vi "Test Executive - 副本.vi"() -> ()   [LabVIEW 2020]
uses:
  Library - Test Executive.llb/Test Executive - Globals.vi
  Library - Test Executive.llb/Test Executive.lvlib
panel:
  in  "Tab Control":T1(tab)
  in  "Serial Number":string
  out "Sequence":string
  out "Report Text":string
  in  "Operator":string
  in  "Save Report":bool
  in  "Clear Report Text":bool
  out "Sequence Name":string="None"
  in  "Abort Button":bool
  in  "Sequence Run":bool
  in  "Sequence Load":bool
  in  "Results Analyser":bool
  in  "Power Down":bool
  in  "Power Up":bool
  in  "Test":u16(ring) items=["1 Current Consumption", "2 Firmware Revision", "3 Indicators", "4 Gain", "5 Sensitivity"]
  in  "Check Test Equipment":bool
  out "errors":errorcluster
  in  "Power Down":bool
  in  "Power Up":bool
  in  "Reset All":bool
  in  "Run Single Test":bool
  out "Help Text":string="This is some help text\n"
  out "Abort":bool
  out "Error":bool
  out "Running":bool
  in  "Quit":bool
  # "Sequence"
  # "Progress"
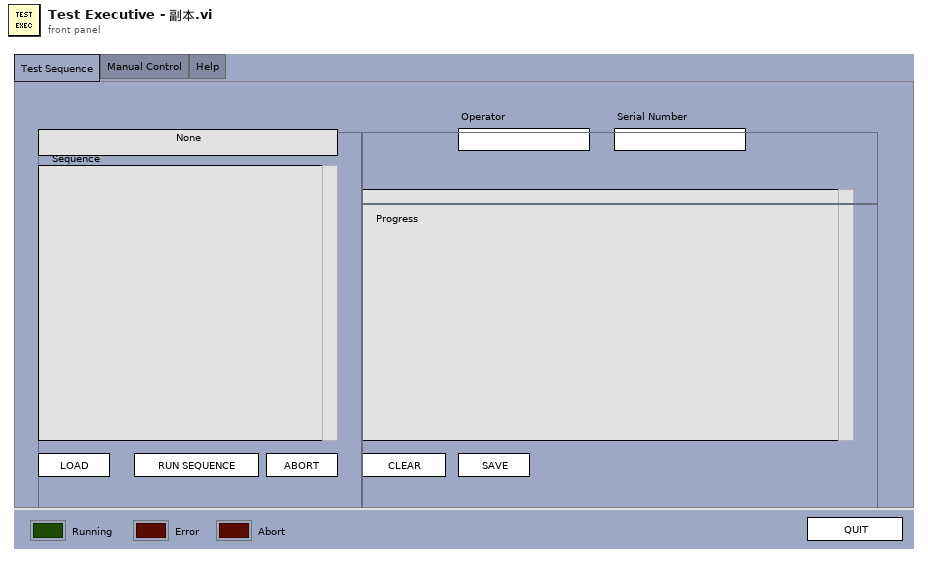
[diagram p1: front panel]
types:
  T1 = enum32{"Test Sequence", "Manual Control", "Help"}
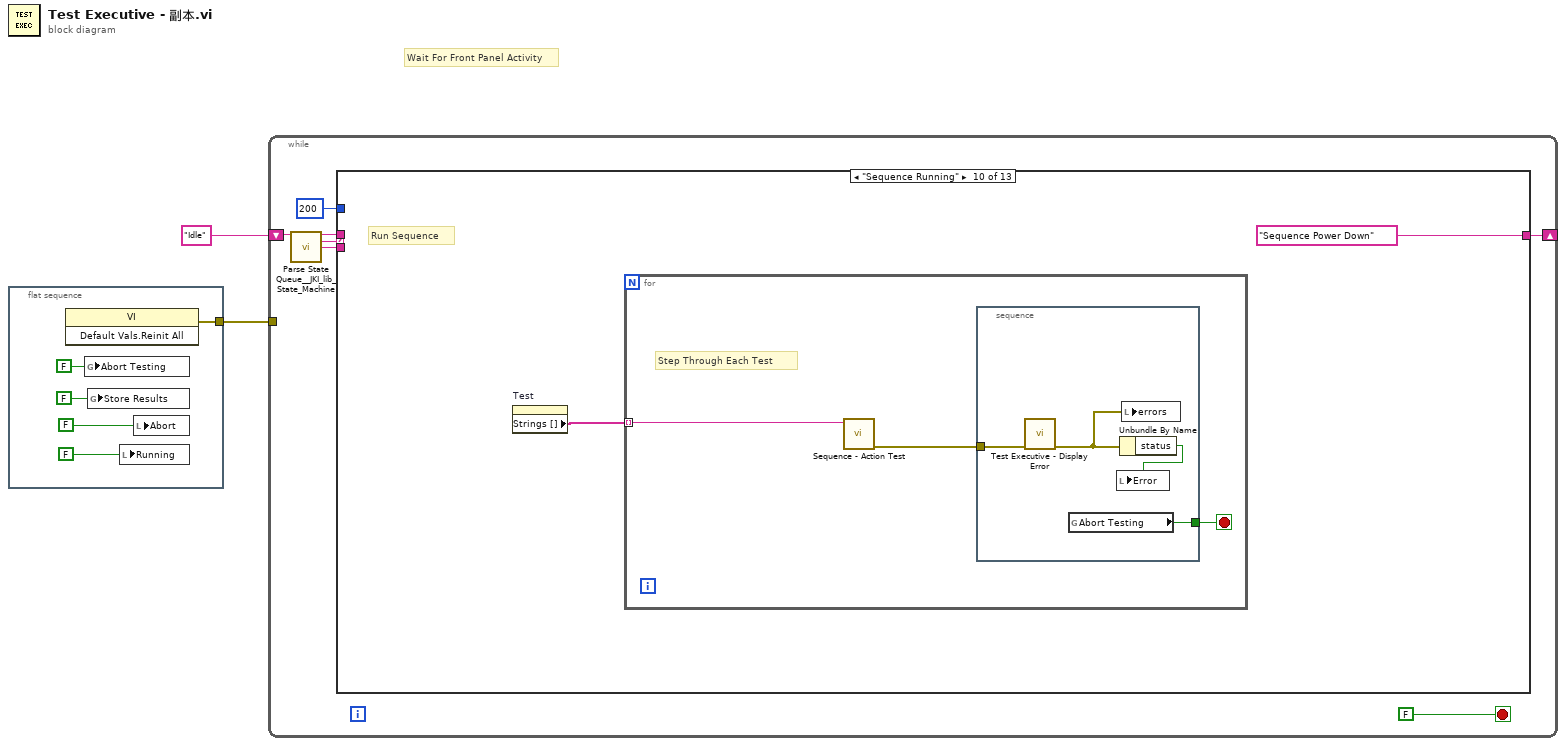
[diagram p0: block diagram]
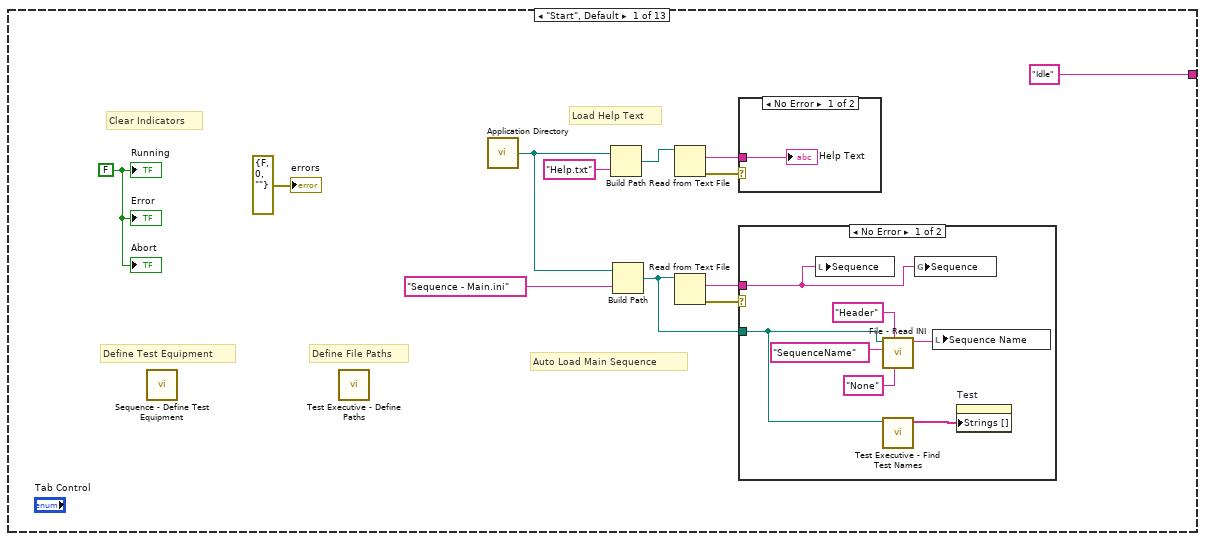
[diagram p2: hidden frame]
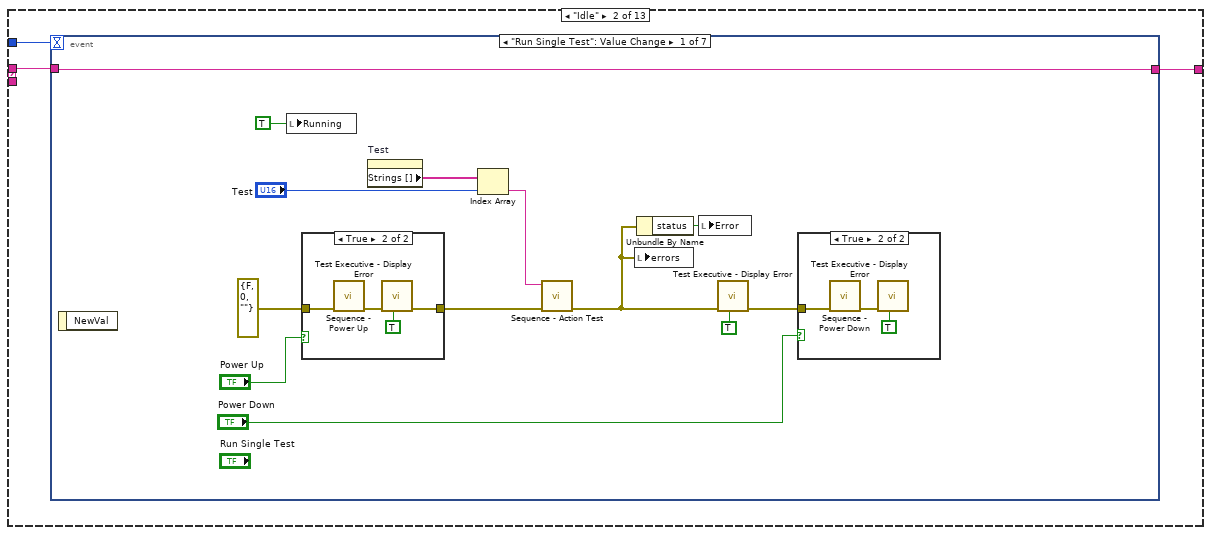
[diagram p5: hidden frame]
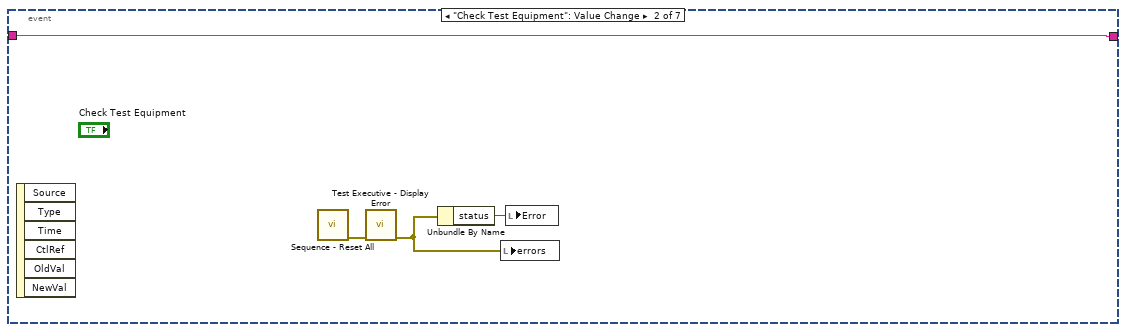
[diagram p8: hidden frame]
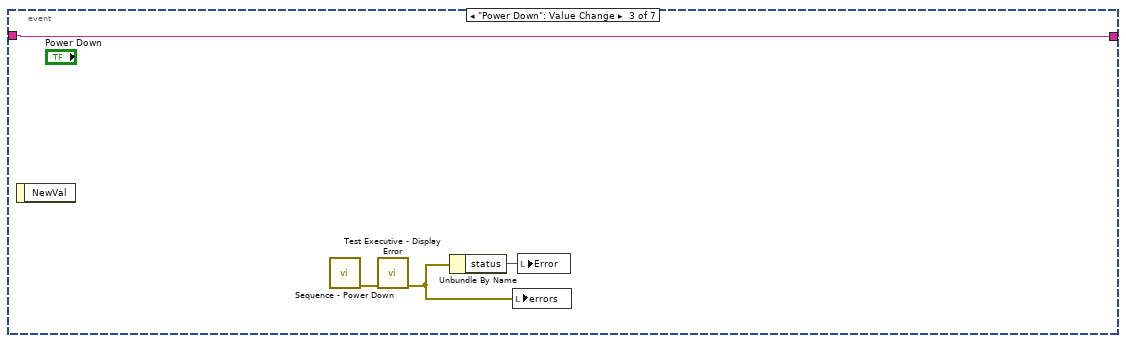
[diagram p9: hidden frame]
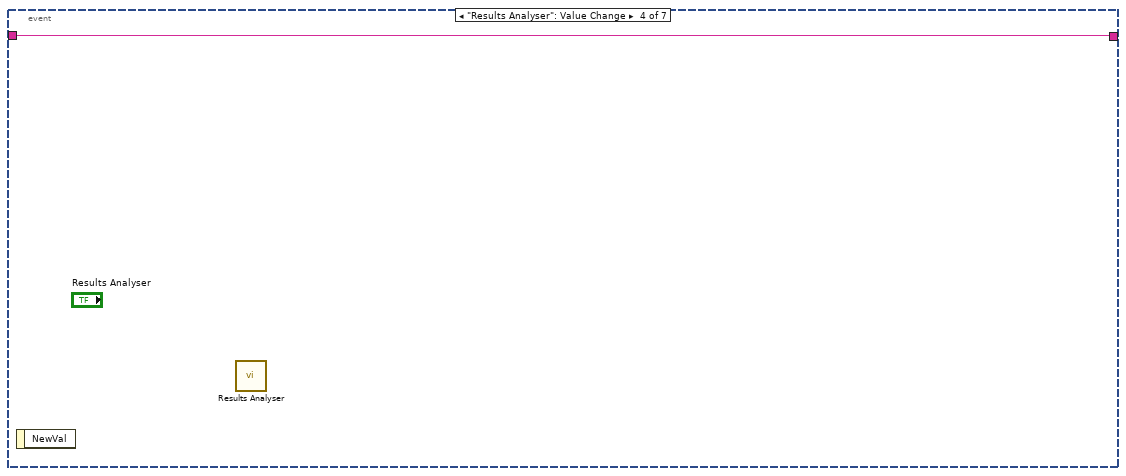
[diagram p10: hidden frame]
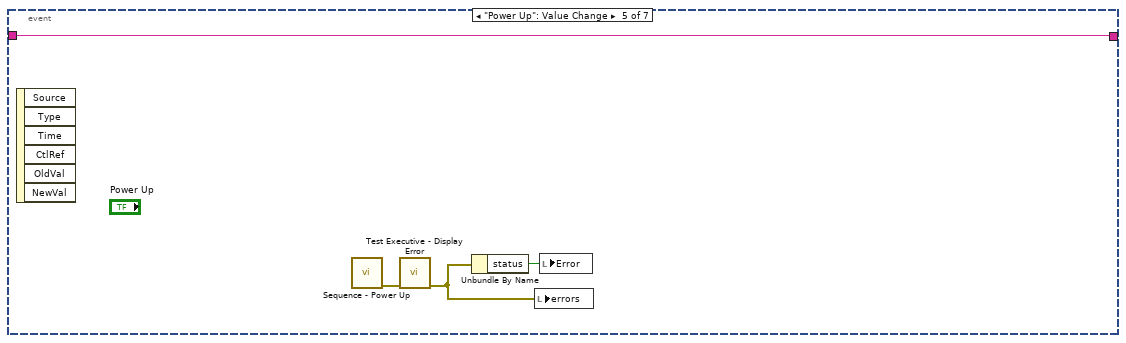
[diagram p11: hidden frame]
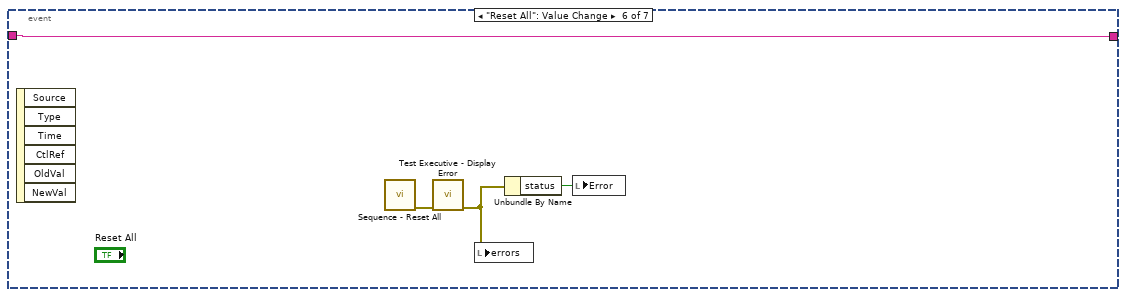
[diagram p12: hidden frame]
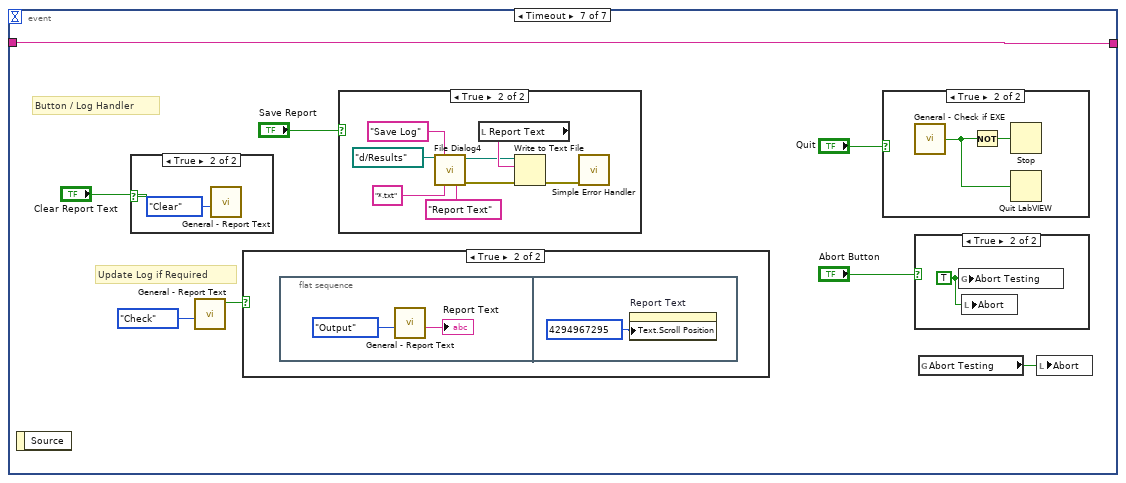
[diagram p13: hidden frame]
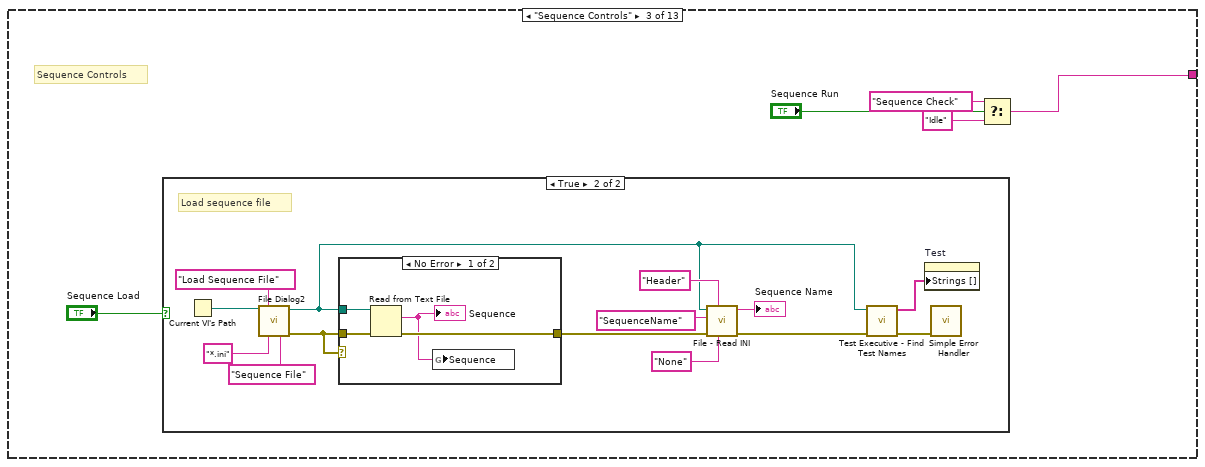
[diagram p19: hidden frame]
diagram:
  # "Wait For Front Panel Activity"
  n1 = flat-sequence {
    tunnel: [w7] -> w2
    frame #0 {
      n2 = invoke class="VI" method="Default Vals.Reinit All"() -> (error out=w7:errorcluster)  [unwired: 3 in, 2 out]
      n3 = global write "Test Executive - Globals.vi" "Abort Testing"(FALSE ("Abort Testing")) -> ()
      n4 = global write "Test Executive - Globals.vi" "Store Results"(FALSE ("Abort Testing")) -> ()
      n5 = local write "Running"(FALSE ("Abort")) -> ()
      n6 = local write "Abort"(FALSE ("Abort")) -> ()
    }
  }
  n7 = while {
    shift-right: [w13] -> _
    shift-left: "Idle" -> [w12]
    tunnel: w2 -> [_]
    stop <- FALSE stop-if-true
    n8 = call <vilib>:"Parse State Queue__JKI_lib_State_Machine.vi"("State Queue"=w12) -> ("Remaining States"=w9:string, "Current State"=w11:string, "Arguments"=w10:string)  [unwired: 12 in]
    n9 = case shown="\"Sequence Running\"" w11 {
      tunnel: ["Idle" w37 w101 w123 w131 w162 "Sequence Pre-Run" ("f") "Sequence Power Up" ("f") "Sequence Running" ("f") "Sequence Power Down" ("f") "Sequence Pass Fail" ("f") "Sequence Store Results" ("f") "Idle" ("f")] -> w13
      tunnel: w10 -> [_ _ _ _ _ _ _ _ _ _ _ _ _]
      tunnel: w9 -> [_ w36 _ _ _ _ _ _ _ _ _ _ _]
      tunnel: 200 -> [_ w35 _ _ _ _ _ _ _ _ _ _ _]
      frame "Start", Default {
        w15 = FALSE ("Running")
        # "Auto Load Main Sequence"
        # "Load Help Text"
        # "Clear Indicators"
        # "Define File Paths"
        # "Define Test Equipment"
        n10 = call "Sequence - Define Test Equipment.vi"() -> ()  [unwired: 11 in, 1 out]
        n11 = call "Test Executive - Define Paths.vi"() -> ()  [unwired: 12 in]
        n12 = call <vilib>:"Application Directory.vi"() -> ("Application Directory"=w16:path)
        n13 = Build Path(base path=w16, name or relative path="Help.txt") -> (appended path=w23:path)
        n14 = Build Path(base path=w16, name or relative path="Sequence - Main.ini") -> (appended path=w17:path)
        n15 = Read from Text File(file (use dialog)=w23) -> (text=w22:string, error out=w21:errorcluster)  [unwired: 3 in, 2 out]
        n16 = Read from Text File(file (use dialog)=w17) -> (text=w19:string, error out=w20:errorcluster)  [unwired: 3 in, 2 out]
        n17 = case shown="No Error" w21 {
          tunnel: w22 -> [w34 _]
          frame No Error {
            "Help Text" <- w34
          }
          frame Error {
          }
        }
        n18 = case shown="No Error" w20 {
          tunnel: w19 -> [w27 _]
          tunnel: w17 -> [w29 _]
          frame No Error {
            n19 = local write "Sequence"(w27) -> ()
            n20 = call "File - Read INI.vi"("Default String"="None", "Section"="Header", "Key"="SequenceName", "configuration file path"=w29) -> ("String"=w30:string)  [unwired: 6 in, 1 out]
            n21 = call "Test Executive - Find Test Names.vi"("Configuration File Path"=w29) -> ("Test Names"=w28:string[])  [unwired: 9 in, 1 out]
            n22 = global write "Test Executive - Globals.vi" "Sequence"(w27) -> ()
            n23 = local write "Sequence Name"(w30) -> ()
            n24 = property on="Test" class="Ring (strict)"("Strings []"=w28) -> ()  [unwired: 2 in, 2 out]
          }
          frame Error {
          }
        }
        "Running" <- w15
        "Error" <- w15
        "errors" <- errorcluster {"status"=FALSE, "code"=0, "source"=""} ("errors")
        "Abort" <- w15
      }
      frame "Idle" {
        n25 = event shown="[0] \"Run Single Test\": Value Change" {
          selector: _ -> [_ _ _ _ _ _ _]
          dyn-events: _ -> [_ _ _ _ _ _ _]
          timeout: w35 -> [_ _ _ _ _ _ _]
          tunnel: [w38 w59 w63 w67 w68 w72 w76] -> w37
          tunnel: w36 -> [w38 w59 w63 w67 w68 w72 w76]
          event "Run Single Test": Value Change {
            n26 = event-data() -> ()  [unwired: 1 in, 1 out]
            n27 = local write "Running"(TRUE ("Running")) -> ()
            n28 = case shown="True" "Power Up" {
              tunnel: errorcluster {"status"=FALSE, "code"=0, "source"=""} ("error in (no error)") -> [w54 w58]
              tunnel: [w54 w57] -> w47
              frame False {
              }
              frame True {
                n29 = call "Sequence - Power Up.vi"("error in (no error)"=w58) -> ("error out"=w56:errorcluster)  [unwired: 10 in]
                n30 = call "Test Executive - Display Error.vi"("Clear Error"=TRUE, "error in (no error)"=w56) -> ("error out"=w57:errorcluster)  [unwired: 9 in]
              }
            }
            n31 = property on="Test" class="Ring (strict)"() -> ("Strings []"=w44:string[])  [unwired: 2 in, 2 out]
            n32 = Index Array(array=w44, index="Test") -> (element=w43:string)
            n33 = call "Sequence - Action Test.vi"("error in (no error)"=w47, "Test"=w43) -> ("error out"=w39:errorcluster)  [unwired: 9 in]
            n34 = local write "errors"(w39) -> ()
            n35 = Unbundle By Name(w39) -> ("status"=w46:bool)
            n36 = local write "Error"(w46) -> ()
            n37 = call "Test Executive - Display Error.vi"("Clear Error"=TRUE, "error in (no error)"=w39) -> ("error out"=w40:errorcluster)  [unwired: 9 in]
            n38 = case shown="True" "Power Down" {
              tunnel: w40 -> [_ w53]
              frame False {
              }
              frame True {
                n39 = call "Sequence - Power Down.vi"("error in (no error)"=w53) -> ("error out"=w52:errorcluster)  [unwired: 10 in]
                n40 = call "Test Executive - Display Error.vi"("Clear Error"=TRUE, "error in (no error)"=w52) -> ()  [unwired: 9 in, 1 out]
              }
            }
          }
          event "Check Test Equipment": Value Change {
            n41 = event-data() -> ()  [unwired: 1 in, 6 out]
            n42 = call "Sequence - Reset All.vi"() -> ("error out"=w61:errorcluster)  [unwired: 11 in]
            n43 = call "Test Executive - Display Error.vi"("error in (no error)"=w61) -> ("error out"=w60:errorcluster)  [unwired: 10 in]
            n44 = Unbundle By Name(w60) -> ("status"=w62:bool)
            n45 = local write "errors"(w60) -> ()
            n46 = local write "Error"(w62) -> ()
          }
          event "Power Down": Value Change {
            n47 = event-data() -> ()  [unwired: 1 in, 1 out]
            n48 = call "Sequence - Power Down.vi"() -> ("error out"=w65:errorcluster)  [unwired: 11 in]
            n49 = call "Test Executive - Display Error.vi"("error in (no error)"=w65) -> ("error out"=w64:errorcluster)  [unwired: 10 in]
            n50 = Unbundle By Name(w64) -> ("status"=w66:bool)
            n51 = local write "errors"(w64) -> ()
            n52 = local write "Error"(w66) -> ()
          }
          event "Results Analyser": Value Change {
            n53 = event-data() -> ()  [unwired: 1 in, 1 out]
            n54 = call "Results Analyser.vi"() -> ()  [unwired: 12 in]
          }
          event "Power Up": Value Change {
            n55 = event-data() -> ()  [unwired: 1 in, 6 out]
            n56 = call "Sequence - Power Up.vi"() -> ("error out"=w70:errorcluster)  [unwired: 11 in]
            n57 = call "Test Executive - Display Error.vi"("error in (no error)"=w70) -> ("error out"=w69:errorcluster)  [unwired: 10 in]
            n58 = Unbundle By Name(w69) -> ("status"=w71:bool)
            n59 = local write "errors"(w69) -> ()
            n60 = local write "Error"(w71) -> ()
          }
          event "Reset All": Value Change {
            n61 = event-data() -> ()  [unwired: 1 in, 6 out]
            n62 = call "Sequence - Reset All.vi"() -> ("error out"=w75:errorcluster)  [unwired: 11 in]
            n63 = call "Test Executive - Display Error.vi"("error in (no error)"=w75) -> ("error out"=w73:errorcluster)  [unwired: 10 in]
            n64 = local write "errors"(w73) -> ()
            n65 = Unbundle By Name(w73) -> ("status"=w74:bool)
            n66 = local write "Error"(w74) -> ()
          }
          event Timeout {
            # "Button / Log Handler"
            # "Update Log if Required"
            n67 = event-data() -> ()  [unwired: 1 in, 1 out]
            n68 = case shown="True" "Clear Report Text" {
              frame False {
              }
              frame True {
                n69 = call "General - Report Text.vi"("Mode (Add)"=enum16{"Add", "Output", "Clear", "Check"}."Clear") -> ()  [unwired: 8 in, 3 out]
              }
            }
            n70 = call "General - Report Text.vi"("Mode (Add)"=enum16{"Add", "Output", "Clear", "Check"}."Check") -> ("Changed Out"=w79:bool)  [unwired: 8 in, 2 out]
            n71 = case shown="True" w79 {
              frame False {
              }
              frame True {
                n72 = flat-sequence {
                  frame #0 {
                    n73 = call "General - Report Text.vi"("Mode (Add)"=enum16{"Add", "Output", "Clear", "Check"}."Output") -> ("Report Text Out"=→"Report Text":string)  [unwired: 8 in, 2 out]
                  }
                  frame #1 {
                    n74 = property on="Report Text" class="Str"("Text.Scroll Position"=u32 4294967295) -> ()  [unwired: 2 in, 2 out]
                  }
                }
              }
            }
            n75 = case shown="True" "Save Report" {
              frame False {
              }
              frame True {
                n76 = call "File Dialog4"("start path"=path "d:/Results", "prompt"="Save Log", "pattern (all files)"="*.txt", "pattern label"="Report Text") -> ("selected path"=w85:path, "error out"=w91:errorcluster)  [unwired: 8 in, 2 out]
                n77 = local read "Report Text"() -> (w90:string)
                n78 = Write to Text File(file (use dialog)=w85, text=w90, error in=w91) -> (error out=w92:errorcluster)  [unwired: 1 in, 2 out]
                n79 = call <vilib>:"Simple Error Handler.vi"("error in (no error)"=w92) -> ()  [unwired: 4 in, 5 out]
              }
            }
            n80 = case shown="True" "Quit" {
              frame False {
              }
              frame True {
                n81 = call "General - Check if EXE.vi"() -> ("EXE"=w94:bool)  [unwired: 2 in]
                n82 = Not(x=w94) -> (.not. x?=w93:bool)
                n83 = Stop(stop? (T)=w93) -> ()
                n84 = Quit LabVIEW(quit? (T)=w94) -> ()
              }
            }
            n85 = case shown="True" "Abort Button" {
              frame False {
              }
              frame True {
                w84 = TRUE ("Abort Testing")
                n86 = global write "Test Executive - Globals.vi" "Abort Testing"(w84) -> ()
                n87 = local write "Abort"(w84) -> ()
              }
            }
            n88 = global read "Test Executive - Globals.vi" "Abort Testing"() -> (w83:bool)
            n89 = local write "Abort"(w83) -> ()
          }
        }
      }
      frame "Sequence Controls" {
        # "Sequence Controls"
        n90 = case shown="True" "Sequence Load" {
          frame False {
          }
          frame True {
            # "Load sequence file"
            n91 = Current VI's Path() -> (path=w115:path)
            n92 = call "File Dialog2"("start path"=w115, "prompt"="Load Sequence File", "pattern (all files)"="*.ini", "pattern label"="Sequence File") -> ("selected path"=w107:path, "error out"=w113:errorcluster)  [unwired: 8 in, 2 out]
            n93 = case shown="No Error" w113 {
              tunnel: w113 -> [w121 w122]
              tunnel: w107 -> [w120 _]
              tunnel: [w119 w122] -> w109
              frame No Error {
                n94 = Read from Text File(file (use dialog)=w120, error in=w121) -> (text=w118:string, error out=w119:errorcluster)  [unwired: 2 in, 2 out]
                "Sequence" <- w118
                n95 = global write "Test Executive - Globals.vi" "Sequence"(w118) -> ()
              }
              frame Error {
              }
            }
            n96 = call "File - Read INI.vi"("Default String"="None", "Section"="Header", "error in (no error)"=w109, "Key"="SequenceName", "configuration file path"=w107) -> ("error out"=w106:errorcluster, "String"=→"Sequence Name":string)  [unwired: 5 in]
            n97 = call "Test Executive - Find Test Names.vi"("error in (no error)"=w106, "Configuration File Path"=w107) -> ("error out"=w105:errorcluster, "Test Names"=w104:string[])  [unwired: 8 in]
            n98 = property on="Test" class="Ring (strict)"("Strings []"=w104) -> ()  [unwired: 2 in, 2 out]
            n99 = call <vilib>:"Simple Error Handler.vi"("error in (no error)"=w105) -> ()  [unwired: 4 in, 5 out]
          }
        }
        n100 = Select(t="Sequence Check", s="Sequence Run", f="Idle") -> (s? t:f=w101:string)
      }
      frame "Sequence Check" {
        # "Check Sequence Name"
        # "Sequence Check"
        n101 = local read "Sequence Name"() -> (w125:string)
        n102 = Equal?(x=w125, y="None") -> (x = y?=w127:bool)
        n103 = case shown="True" w127 {
          tunnel: "Sequence Start" -> [w128 _]
          tunnel: [w128 "Idle"] -> w123
          frame False {
          }
          frame True {
            n104 = call "Dialog Box - One Button.vi"("Text"="ERROR: Sequence name is set to \"None\".") -> ()  [unwired: 10 in, 1 out]
          }
        }
      }
      frame "Sequence Start" {
        # "Enter Serial Number"
        # "Enter Operator Name"
        # "Start of Sequence"
        # "Configure Results Storage"
        n105 = local read "Operator"() -> (w147:string)
        n106 = call <vilib>:"Dflt Data Dir.vi"() -> ("App:Default Data Directory"=w135:path)
        n107 = call "Dialog Box - Text Input.vi"("Value In"=w147, "Text"="Please enter your name") -> ("error out"=w150:errorcluster, "Value Out"=w140:string)  [unwired: 8 in]
        n108 = Build Path(base path=w135, name or relative path="Results") -> (appended path=w137:path)
        n109 = call "General - Check if Mac.vi"() -> ("Mac"=w138:bool)  [unwired: 2 in]
        n110 = Path To String(path=w137) -> (string=w136:string)
        n111 = local write "Operator"(w140) -> ()
        n112 = global write "Test Executive - Globals.vi" "Operator Name"(w140) -> ()
        n113 = case shown="True" w138 {
          tunnel: [w156 w160] -> w143
          tunnel: w136 -> [w154 w158]
          frame True {
            n114 = call "Test Executive - Sequence File Value.vi"("Default String"=w154, "Section (Current Test)"="results" ("Section"), "Key"="directorymac") -> ("String"=w156:string)  [unwired: 5 in, 3 out]
          }
          frame False {
            n115 = call "Test Executive - Sequence File Value.vi"("Default String"=w158, "Section (Current Test)"="results" ("Section"), "Key"="directorywin") -> ("String"=w160:string)  [unwired: 5 in, 3 out]
          }
        }
        n116 = local read "Serial Number"() -> (w148:string)
        n117 = String To Path(string=w143) -> (path=w141:path)
        n118 = global write "Test Executive - Globals.vi" "Results Directory"(w141) -> ()
        n119 = call "Results Storage - Setup.vi"("Rename Files on Close"=TRUE, "Results Directory"=w141) -> ()  [unwired: 9 in, 1 out]
        n120 = call "Dialog Box - Text Input.vi"("error in (no error)"=w150, "Value In"=w148, "Text"="Please enter serial number") -> ("Value Out"=w133:string)  [unwired: 7 in, 1 out]
        n121 = Empty String/Path?(string/path=w133) -> (empty?=w132:bool)
        n122 = local write "Serial Number"(w133) -> ()
        n123 = global write "Test Executive - Globals.vi" "Serial Number"(w133) -> ()
        n124 = case shown="False" w132 {
          tunnel: ["Sequence Check Equipment" ("f") "Idle" ("f")] -> w131
          frame False {
          }
          frame True {
            n125 = call "Dialog Box - One Button.vi"("Text"="ERROR: Serial number cannot be blank.") -> ()  [unwired: 10 in, 1 out]
          }
        }
        n126 = global write "Test Executive - Globals.vi" "Abort Testing"(FALSE ("Abort Testing")) -> ()
        n127 = global write "Test Executive - Globals.vi" "Unit Passed"(FALSE ("Pass")) -> ()
        n128 = call "General - Report Text.vi"("Mode (Add)"=enum16{"Add", "Output", "Clear", "Check"}."Clear") -> ()  [unwired: 8 in, 3 out]
      }
      frame "Sequence Check Equipment" {
        # "Check Test Equipment"
        # "Check Test Equipment"
        n129 = call "Sequence - Check Test Equipment.vi"() -> ("error out"=w165:errorcluster, "PASS"=w166:bool)  [unwired: 10 in]
        n130 = Not(x=w166) -> (.not. x?=w164:bool)
        n131 = case shown="True" w164 {
          tunnel: "Sequence Asset" -> [w167 _]
          tunnel: [w167 "Idle"] -> w162
          tunnel: w165 -> [_ _]
          frame False {
          }
          frame True {
            n132 = call "Dialog Box - One Button.vi"("Text"="ERROR: Test equipment check failed.") -> ()  [unwired: 10 in, 1 out]
          }
        }
      }
      frame "Sequence Asset" {
        # "Test Equipment is Defined is \"Sequence - Define Test Equipment.vi\""
        # "Enter Equipment Asset Numbers"
        n133 = global read "Test Executive - Globals.vi" "Asset Number Recording"() -> (w170:bool)
        n134 = case shown="True" w170 {
          frame False {
          }
          frame True {
            n135 = call "Test Equipment - Asset Numbers.vi"("Mode"=enum16{"Edit", "Define", "Load", "Save", "CSV"}."Load") -> ("error out"=w172:errorcluster)  [unwired: 9 in, 1 out]
            n136 = call "Test Equipment - Asset Numbers.vi"("error in (no error)"=w172, "Mode"=enum16{"Edit", "Define", "Load", "Save", "CSV"}."Edit") -> ("error out"=w173:errorcluster)  [unwired: 8 in, 1 out]
            n137 = call "Test Equipment - Asset Numbers.vi"("error in (no error)"=w173, "Mode"=enum16{"Edit", "Define", "Load", "Save", "CSV"}."Save") -> ()  [unwired: 8 in, 2 out]
          }
        }
      }
      frame "Sequence Pre-Run" {
        # "Create Results File"
        # "Record Serial Number and Operator Name"
        # "Record Start Time"
        # "Start Sequence"
        n138 = call "General - Start Stop Time.vi"("Start / Stop (Start)"=enum16{"Start", "Stop"}."Start", "Initial String"="Sequence Started") -> ("String with Time / Date"=w191:string)  [unwired: 8 in, 1 out]
        n139 = local write "Running"(TRUE ("Test Running")) -> ()
        n140 = call "General - Report Text.vi"("Mode (Add)"=enum16{"Add", "Output", "Clear", "Check"}."Add", "Text In"=w191) -> ("error out"=w182:errorcluster)  [unwired: 7 in, 2 out]
        n141 = Concatenate Strings("Serial Number: " ("string"), "Serial Number") -> (w187:string)
        n142 = call "General - Report Text.vi"("error in (no error)"=w182, "Mode (Add)"=enum16{"Add", "Output", "Clear", "Check"}."Add", "Text In"=w187) -> ("error out"=w181:errorcluster)  [unwired: 6 in, 2 out]
        n143 = global write "Test Executive - Globals.vi" "Store Results"(TRUE ("Store Results")) -> ()
        n144 = Concatenate Strings("Operator Name: " ("string"), "Operator") -> (w184:string)
        n145 = call "Results Storage - Create Results File.vi"("Operator Name"="Operator", "Serial Number"="Serial Number") -> ()  [unwired: 9 in, 1 out]
        n146 = call "General - Report Text.vi"("error in (no error)"=w181, "Mode (Add)"=enum16{"Add", "Output", "Clear", "Check"}."Add", "Text In"=w184) -> ()  [unwired: 6 in, 3 out]
      }
      frame "Sequence Power Up" {
        # "Reset all Test Equipment then Power Up Unit Under Test"
        # "Sequence Power Up"
        n147 = call "Sequence - Reset All.vi"() -> ("error out"=w198:errorcluster)  [unwired: 11 in]
        n148 = call "Test Executive - Display Error.vi"("Clear Error"=TRUE, "error in (no error)"=w198) -> ("error out"=w197:errorcluster)  [unwired: 9 in]
        n149 = call "Sequence - Power Up.vi"("error in (no error)"=w197) -> ("error out"=w196:errorcluster)  [unwired: 10 in]
        n150 = call "Test Executive - Display Error.vi"("Clear Error"=TRUE, "error in (no error)"=w196) -> ()  [unwired: 9 in, 1 out]
      }
      frame "Sequence Running" {
        # "Run Sequence"
        n151 = property on="Test" class="Ring (strict)"() -> ("Strings []"=w200:string[])  [unwired: 2 in, 2 out]
        n152 = for {
          tunnel: w200 -> [w203] mode=indexing
          stop <- w204 stop-if-true
          # "Step Through Each Test"
          n153 = call "Sequence - Action Test.vi"("Test"=w203) -> ("error out"=w202:errorcluster)  [unwired: 10 in]
          n154 = stacked-sequence {
            tunnel: [w207] -> w204
            tunnel: w202 -> [w206]
            frame #0 {
              n155 = call "Test Executive - Display Error.vi"("error in (no error)"=w206) -> ("error out"=w205:errorcluster)  [unwired: 10 in]
              n156 = global read "Test Executive - Globals.vi" "Abort Testing"() -> (w207:bool)
              n157 = Unbundle By Name(w205) -> ("status"=w208:bool)
              n158 = local write "Error"(w208) -> ()
              n159 = local write "errors"(w205) -> ()
            }
          }
        }
      }
      frame "Sequence Power Down" {
        # "Power Down Unit Under Test then Reset all Test Equipment"
        # "Sequence Power Down"
        n160 = call "Sequence - Power Down.vi"() -> ("error out"=w209:errorcluster)  [unwired: 11 in]
        n161 = call "Test Executive - Display Error.vi"("Clear Error"=TRUE, "error in (no error)"=w209) -> ("error out"=w210:errorcluster)  [unwired: 9 in]
        n162 = call "Sequence - Reset All.vi"("error in (no error)"=w210) -> ("error out"=w211:errorcluster)  [unwired: 10 in]
        n163 = call "Test Executive - Display Error.vi"("Clear Error"=TRUE, "error in (no error)"=w211) -> ()  [unwired: 9 in, 1 out]
      }
      frame "Sequence Pass Fail" {
        # "Add Stop Time"
        # "Sequence Pass / Fail"
        # "Display Banner"
        # "Pass / Fail ??"
        n164 = call "General - Report Text.vi"("Mode (Add)"=enum16{"Add", "Output", "Clear", "Check"}."Output") -> ("Report Text Out"=w224:string)  [unwired: 8 in, 2 out]
        n165 = Search/Split String(string=w224, search string/char (-)="ERROR") -> (offset of match=w244:i32)  [unwired: 1 in, 2 out]
        n166 = Search/Split String(string=w224, search string/char (-)="FAIL") -> (offset of match=w238:i32)  [unwired: 1 in, 2 out]
        n167 = Search/Split String(string=w224, search string/char (-)="PASS") -> (offset of match=w225:i32)  [unwired: 1 in, 2 out]
        n168 = Greater Than 0?(x=w244) -> (x > 0?=w245:bool)
        n169 = Greater Than 0?(x=w238) -> (x > 0?=w239:bool)
        n170 = Greater Than 0?(x=w225) -> (x > 0?=w222:bool)
        n171 = Select(t="UNIT PASSED", s=w222, f="UNIT FAILED") -> (s? t:f=w221:string)
        n172 = Select(t="UNIT FAILED", s=w239, f=w221) -> (s? t:f=w246:string)
        n173 = Select(t="UNIT FAILED (ERRORS)", s=w245, f=w246) -> (s? t:f=w219:string)
        n174 = global read "Test Executive - Globals.vi" "Abort Testing"() -> (w216:bool)
        n175 = Select(t="TESTING ABORTED", s=w216, f=w219) -> (s? t:f=w217:string)
        n176 = Select(t="Sequence Aborted", s=w216, f="Sequence Completed" ("Initial String")) -> (s? t:f=w233:string)
        n177 = call "General - Report Text.vi"("Mode (Add)"=enum16{"Add", "Output", "Clear", "Check"}."Add", "Text In"=w217) -> ("error out"=w229:errorcluster)  [unwired: 7 in, 2 out]
        n178 = call "General - Start Stop Time.vi"("Start / Stop (Start)"=enum16{"Start", "Stop"}."Stop", "Initial String"=w233) -> ("String with Time / Date"=w231:string)  [unwired: 8 in, 1 out]
        n179 = Equal?(x="UNIT PASSED", y=w217) -> (x = y?=w215:bool)
        n180 = global write "Test Executive - Globals.vi" "Unit Passed"(w215) -> ()
        n181 = call "Dialog Box - Pass Fail Banner.vi"("Pass"=w215, "Text"=w217) -> ()  [unwired: 9 in, 1 out]
        n182 = call "General - Report Text.vi"("error in (no error)"=w229, "Mode (Add)"=enum16{"Add", "Output", "Clear", "Check"}."Add", "Text In"=w231) -> ()  [unwired: 6 in, 3 out]
      }
      frame "Sequence Store Results" {
        # "Record Asset Numbers"
        # "Sequence Store Results"
        # "Close Results File"
        n183 = global read "Test Executive - Globals.vi" "Asset Number Recording"() -> (w250:bool)
        n184 = global read "Test Executive - Globals.vi" "Unit Passed"() -> (w247:bool)
        n185 = case shown="True" w250 {
          tunnel: [_ w258] -> w249
          frame False {
          }
          frame True {
            n186 = call "Test Equipment - Asset Numbers.vi"("Mode"=enum16{"Edit", "Define", "Load", "Save", "CSV"}."CSV") -> ("Output"=w259:string)  [unwired: 9 in, 1 out]
            n187 = call "Results Storage - Add Text.vi"("Add New Line (True)"=FALSE, "Text"=w259) -> ("error out"=w258:errorcluster)  [unwired: 9 in]
          }
        }
        n188 = global read "Test Executive - Globals.vi" "Abort Testing"() -> (w248:bool)
        n189 = Select(t=enum16{"auto", "passed", "failed", "aborted"}."passed" ("Result (auto)"), s=w247, f=enum16{"auto", "passed", "failed", "aborted"}."failed" ("Result (auto)")) -> (s? t:f=w252:enum16{"auto", "passed", "failed", "aborted"})
        n190 = Select(t=enum16{"auto", "passed", "failed", "aborted"}."aborted" ("Result (auto)"), s=w248, f=w252) -> (s? t:f=w251:enum16{"auto", "passed", "failed", "aborted"})
        n191 = call "Results Storage - Close Results File.vi"("error in (no error)"=w249, "Result (auto)"=w251) -> ()  [unwired: 9 in, 1 out]
      }
    }
  }
